vi "Shuffle.vi"(8 "error in (no error)":errorcluster, 10 "North":enum16{"North", "Eeast", "South", "West"}(ring), 11 "Proto in":refnum<class "Board.lvclass">) -> (0 "error out":errorcluster, 3 "Proto out":refnum<class "Board.lvclass">)   [LabVIEW 2021, in "Board.lvclass"]
uses:
  Board.lvclass
  Board.lvclass/Board.ctl
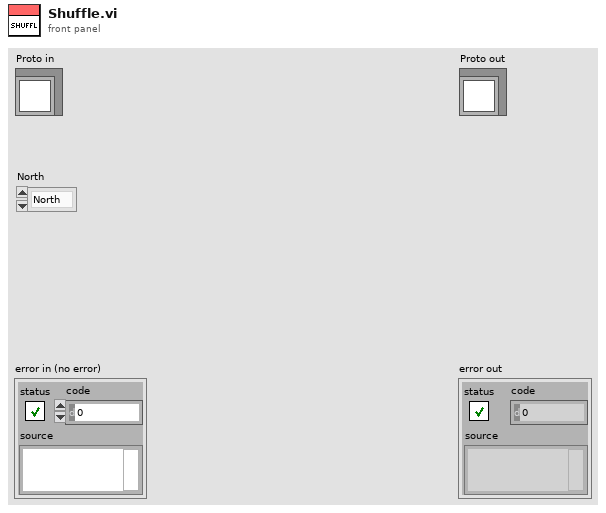
[diagram p1: front panel]
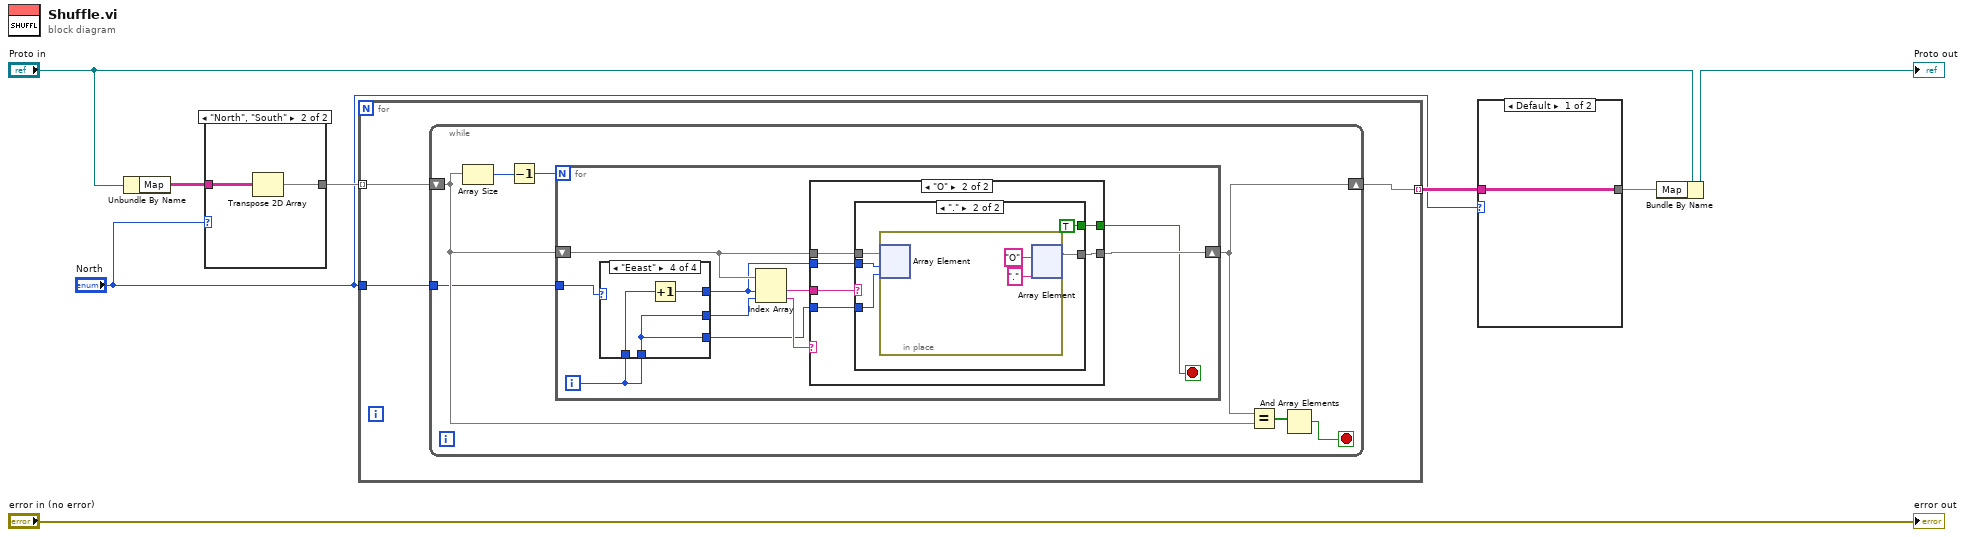
[diagram p0: block diagram]
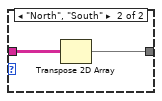
[diagram p2: hidden frame]
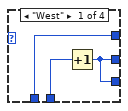
[diagram p4: hidden frame]
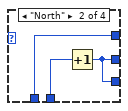
[diagram p5: hidden frame]
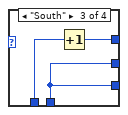
[diagram p6: hidden frame]
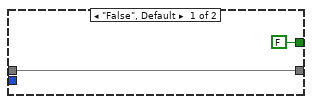
[diagram p7: hidden frame]
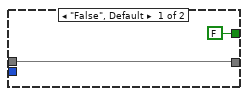
[diagram p8: hidden frame]
diagram:
  n1 = Unbundle By Name("Proto in") -> ("Map"=w6:string[][])
  n2 = case shown="\"North\", \"South\"" "North" {
    tunnel: w6 -> [w9 w11]
    tunnel: [w9 w10] -> w4
    frame Default {
    }
    frame "North", "South" {
      n3 = Transpose 2D Array(2D array=w11) -> (transposed array=w10:string[][])
    }
  }
  n4 = for {
    tunnel: w4 -> [w14] mode=indexing
    tunnel: [w13] -> w3 mode=indexing
    tunnel: "North" -> [w12]
    n5 = while {
      shift-right: [w16] -> w13
      shift-left: w14 -> [w19]
      tunnel: w12 -> [w15]
      stop <- w17 stop-if-true
      n6 = Array Size(array=w19) -> (size(s)=w21:i32)
      n7 = Decrement(x=w21) -> (x-1=w20:i32)
      n8 = for {
        N: w20 -> [_]
        shift-right: [w27] -> w16
        shift-left: w19 -> [w29]
        tunnel: w15 -> [w25]
        i -> [w23]
        stop <- w26 stop-if-true
        n9 = case shown="\"Eeast\"" w25 {
          tunnel: [w33 w37 w38 w41] -> w28
          tunnel: w23 -> [w33 w37 w40 w43]
          tunnel: [w32 w35 w39 w42] -> w24
          tunnel: w23 -> [w34 w36 w39 w42]
          tunnel: [w32 w35 w39 w42] -> w22
          frame "West" {
            n10 = Increment(x=w34) -> (x+1=w32:i32)
          }
          frame "North" {
            n11 = Increment(x=w36) -> (x+1=w35:i32)
          }
          frame "South" {
            n12 = Increment(x=w40) -> (x+1=w38:i32)
          }
          frame "Eeast" {
            n13 = Increment(x=w43) -> (x+1=w41:i32)
          }
        }
        n14 = Index Array(array=w29, index #1=w28, index #2=w24) -> (element #1=w30:string, element #2=w31:string)
        n15 = case shown="\"O\"" w31 {
          tunnel: w30 -> [_ w50]
          tunnel: w29 -> [w45 w51]
          tunnel: w28 -> [_ w49]
          tunnel: w22 -> [_ w48]
          tunnel: [w45 w47] -> w27
          tunnel: [FALSE w46] -> w26
          frame "False", Default {
          }
          frame "O" {
            n16 = case shown="\".\"" w50 {
              tunnel: w51 -> [w53 w58]
              tunnel: w49 -> [_ w57]
              tunnel: w48 -> [_ w56]
              tunnel: [w53 w55] -> w47
              tunnel: [FALSE TRUE] -> w46
              frame "False", Default {
              }
              frame "." {
                n17 = in-place {
                  n18 = in-place-array #1(w58, w57, w56) -> ()  [unwired: 2 out]
                  n19 = in-place-array #1("O" ("element"), "." ("element")) -> (w55:string[])  [unwired: 2 out]
                }
              }
            }
          }
        }
      }
      n20 = Equal?(x=w16, y=w19) -> (x = y?=w18:bool[])
      n21 = And Array Elements(Boolean array=w18) -> (logical AND=w17:bool)
    }
  }
  n22 = case shown="Default" "North" {
    tunnel: w3 -> [w61 w63]
    tunnel: [w61 w62] -> w2
    frame Default {
    }
    frame "North", "South" {
      n23 = Transpose 2D Array(2D array=w63) -> (transposed array=w62:string[][])
    }
  }
  n24 = Bundle By Name(cluster="Proto in", "Map"=w2) -> (→"Proto out":refnum<class "Board.lvclass">)
  "error out" <- "error in (no error)"
